vi "Event Handle Loop_Close Page Event.vi"(8 "error in (no error)":errorcluster, 10 "Label":string, 11 "QTab Class in":refnum<class "QTab Class.lvclass">) -> (0 "error out":errorcluster, 2 "Confirm":bool, 3 "QTab Class out":refnum<class "QTab Class.lvclass">)   [LabVIEW 2020, in "QTab.lvlib" / "QTab Class.lvclass"]
uses:
  QTab Class.lvclass
  QTab Class.lvclass/QTab Class.ctl
  Close Event Data.ctl
  <vilib>/Utility/miscctls.llb/LVMapReplaceAction.ctl
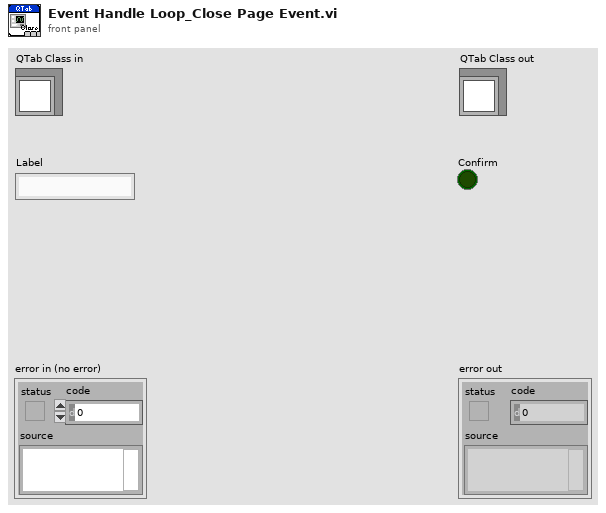
[diagram p1: front panel]
types:
  T1 = typedef "LVMapReplaceAction.ctl" = enum32{"Modify Entry only if found", "Add or Modify Entry", "Delete Entry"}
  T2 = typedef "QTab.lvlib/QTab Class.lvclass/Close Event Data.ctl" = cluster{"VI Refnum":refnum<vi>, "Page Name":string, "Confirm Notifier":refnum<notifier>}
  T3 = typedef "QTab.lvlib/QTab Class.lvclass/Pag Attribute.ctl" = cluster{"VI Refnum":refnum<vi>, "Page Name":string, "Closeable":bool, "Draggable":bool, "Pop-Out":bool}
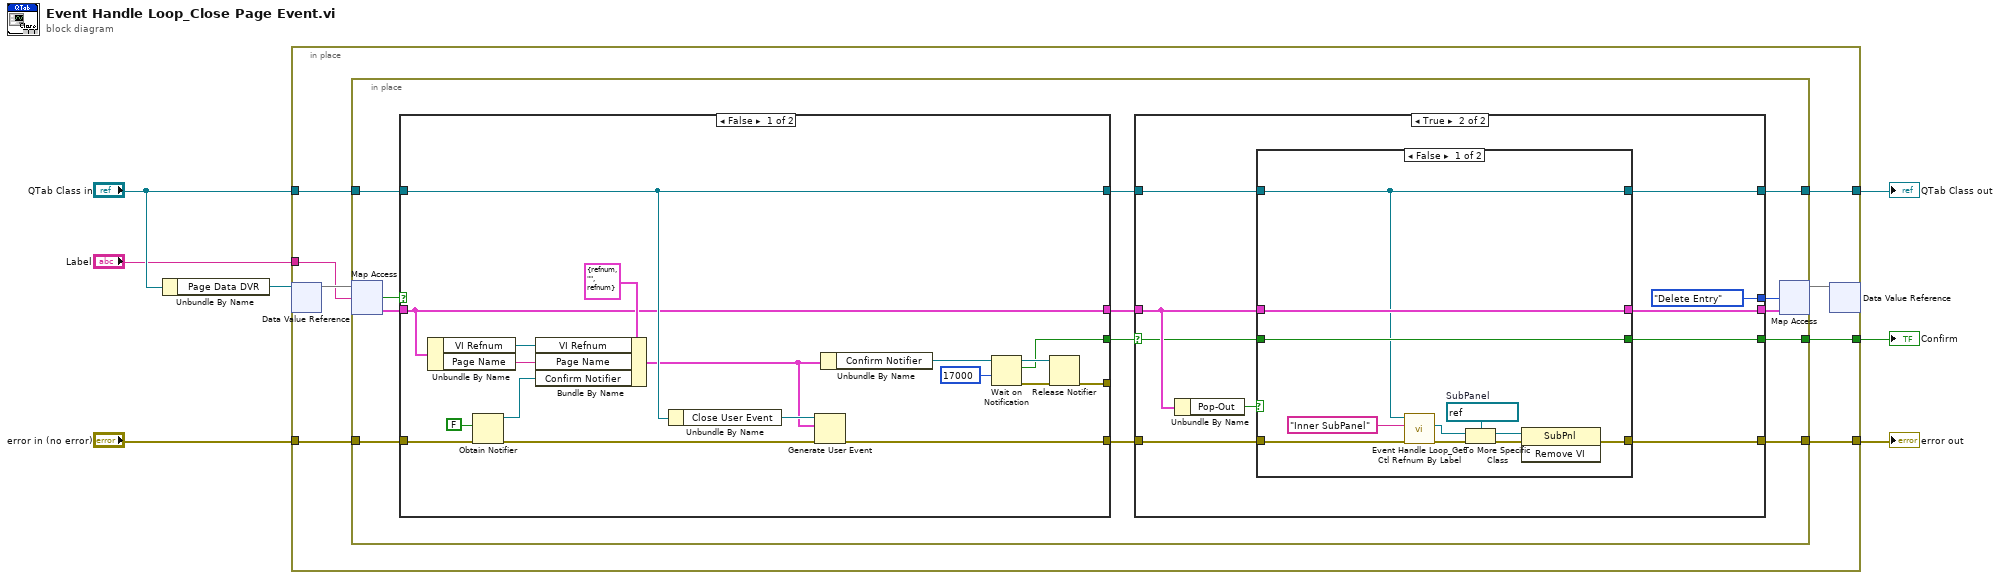
[diagram p0: block diagram]
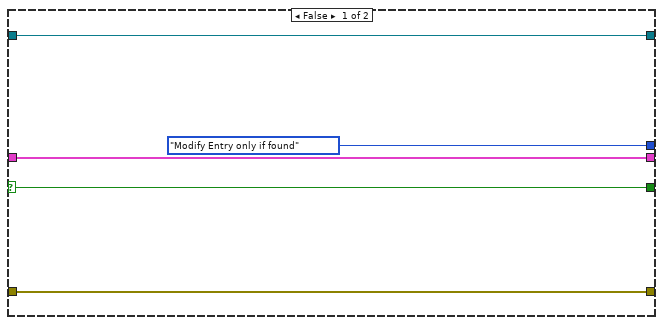
[diagram p2: hidden frame]
diagram:
  n1 = Unbundle By Name("QTab Class in") -> ("Page Data DVR"=w3:refnum<data-value>)
  n2 = in-place {
    in-place-border: [w15] -> w7
    in-place-border: [w14] -> w6
    in-place-border: "QTab Class in" -> [w13]
    in-place-border: "error in (no error)" -> [w12]
    in-place-border: "Label" -> [w10]
    in-place-border: [w8] -> w1
    n3 = in-place-dvr #1(w3) -> (w11:map{string, T3})  [unwired: 1 out]
    n4 = in-place {
      in-place-border: [w25] -> w15
      in-place-border: [w24] -> w14
      in-place-border: w13 -> [w23]
      in-place-border: w12 -> [w22]
      in-place-border: [w16] -> w8
      n5 = in-place-map #2(w11, w10) -> (w20:T3, w21:bool)  [unwired: 1 in]
      n6 = case shown="False" w21 {
        tunnel: w23 -> [w70 w79]
        tunnel: w22 -> [w73 w78]
        tunnel: [w70 w79] -> w26
        tunnel: [w66 w78] -> w28
        tunnel: [w62 _] -> _
        tunnel: [w60 _] -> w27
        tunnel: w20 -> [w59 w77]
        tunnel: [w59 w77] -> w18
        frame False {
          n7 = Unbundle By Name(w59) -> ("VI Refnum"=w75:refnum<vi>, "Page Name"=w74:string)
          n8 = Obtain Notifier(notification data type=FALSE, error in (no error)=w73) -> (notifier out=w71:refnum<notifier>, error out=w69:errorcluster)  [unwired: 2 in, 1 out]
          n9 = Bundle By Name(cluster=T2 {"VI Refnum"=refnum, "Page Name"="", "Confirm Notifier"=refnum} ("Close Event Data"), "VI Refnum"=w75, "Page Name"=w74, "Confirm Notifier"=w71) -> (w67:T2)
          n10 = Unbundle By Name(w70) -> ("Close User Event"=w68:refnum<user-event>)
          n11 = Generate User Event(user event=w68, event data cluster=w67, error in=w69) -> (error out=w66:errorcluster)  [unwired: 1 in, 1 out]
          n12 = Unbundle By Name(w67) -> ("Confirm Notifier"=w65:refnum<notifier>)
          n13 = Wait on Notification(notifier=w65, timeout in ms (-1)=17000) -> (notifier out=w64:refnum<notifier>, notification=w60:bool, error out=w63:errorcluster)  [unwired: 2 in, 1 out]
          n14 = Release Notifier(notifier=w64, error in (no error)=w63) -> (error out=w62:errorcluster)  [unwired: 1 in, 2 out]
        }
        frame True {
        }
      }
      n15 = case shown="True" w27 {
        selector: w27 -> [w32 w36]
        tunnel: w28 -> [w31 w43]
        tunnel: w26 -> [w33 w40]
        tunnel: [w33 w39] -> w25
        tunnel: [w32 w35] -> w16
        tunnel: [w31 w42] -> w24
        tunnel: [LVMapReplaceAction."Modify Entry only if found" ("action") LVMapReplaceAction."Delete Entry" ("action")] -> w19
        tunnel: w18 -> [w29 w37]
        tunnel: [w29 w34] -> w17
        frame False {
        }
        frame True {
          n16 = Unbundle By Name(w37) -> ("Pop-Out"=w38:bool)
          n17 = case shown="False" w38 {
            tunnel: w43 -> [w48 w58]
            tunnel: [w47 w58] -> w42
            tunnel: w40 -> [w44 w55]
            tunnel: [w44 w55] -> w39
            tunnel: w37 -> [w45 w56]
            tunnel: w36 -> [w46 w57]
            tunnel: [w46 w57] -> w35
            tunnel: [w45 w56] -> w34
            frame False {
              w51 = refnum<vi> refnum  # SubPanel
              n18 = call "Event Handle Loop_Get Ctl Refnum By Label.vi"("error in (no error)"=w48, "Label"="Inner SubPanel", "QTab Class in"=w44) -> ("error out"=w53:errorcluster, "Ctl Refnum"=w52:refnum<vi>)  [unwired: 6 in, 1 out]
              n19 = To More Specific Class(target class=w51, reference=w52, error in=w53) -> (specific class reference=w49:refnum<vi>, error out=w50:errorcluster)
              n20 = invoke class="SubPnl" method="Remove VI"(reference=w49, error in=w50) -> (error out=w47:errorcluster)  [unwired: 1 in, 2 out]
            }
            frame True {
            }
          }
        }
      }
      n21 = in-place-map #2(w17, w19) -> (w9:map{string, T3})  [unwired: 2 out]
    }
    n22 = in-place-dvr #1(w9) -> ()  [unwired: 2 out]
  }
  "error out" <- w6
  "QTab Class out" <- w7
  "Confirm" <- w1
